vi "E Save as.vi"(0 "Excel._WorkBook":refnum<k7>, 5 "File path/保存路径":path, 7 "File path/保存名称":string, 11 "error in (no error)":errorcluster) -> (15 "error out":errorcluster)   [LabVIEW 2011]
doc: "将表格按指定的名称另存在指定的路径下并关闭此表格。"
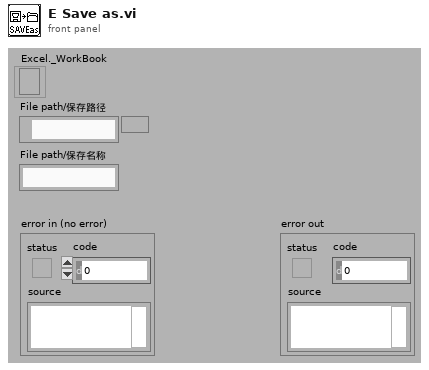
[diagram p1: front panel]
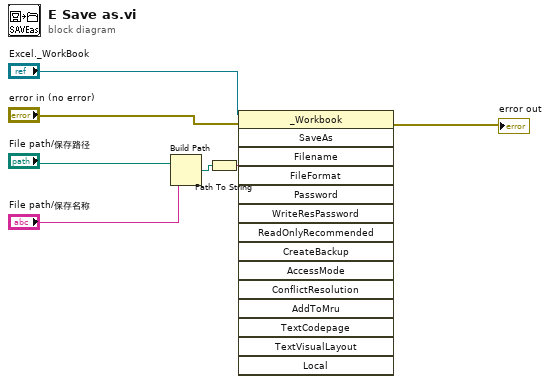
[diagram p0: block diagram]
diagram:
  n1 = Build Path(base path="File path/保存路径", name or relative path="File path/保存名称") -> (appended path=w5:path)
  n2 = Path To String(path=w5) -> (string=w4:string)
  n3 = invoke class="_Workbook" method="SaveAs"(reference="Excel._WorkBook", error in="error in (no error)", "Filename"=w4) -> (error out=→"error out":errorcluster)  [unwired: 12 in, 14 out]
